vi "OpenDevices.vi"(7 "error In":errorcluster, 10 "Names":string[](array[string])) -> (0 "error out":errorcluster, 2 "Serial nos":u32[](array[numeric]), 3 "IDs":i32[](array[numeric]))   [LabVIEW 2020]
uses:
  libximc.lvlib
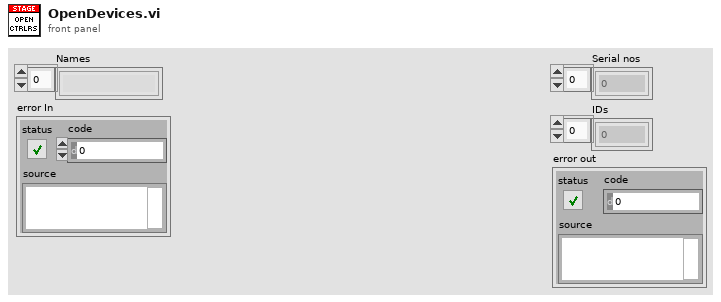
[diagram p1: front panel]
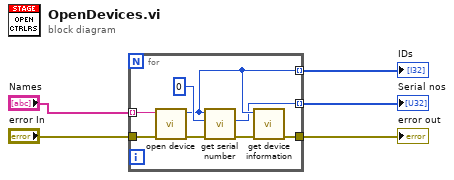
[diagram p0: block diagram]
diagram:
  n1 = for {
    tunnel: "error In" -> [w13]
    tunnel: [w6] -> w1
    tunnel: [w10] -> w2 mode=indexing
    tunnel: "Names" -> [w8] mode=indexing
    tunnel: [w7] -> w3 mode=indexing
    n2 = call "open device.vi"("error in (no error)"=w13, "uri"=w8) -> ("error out"=w9:errorcluster, "function return"=w10:i32)  [unwired: 8 in]
    n3 = call "get serial number.vi"("error in (no error)"=w9, "SerialNumber"=u32 0 ("serial"), "id"=w10) -> ("error out"=w11:errorcluster, "SerialNumber out"=w7:u32)  [unwired: 6 in, 1 out]
    n4 = call "get device information.vi"("error in (no error)"=w11, "id"=w10) -> ("error out"=w6:errorcluster)  [unwired: 7 in, 2 out]
  }
  "Serial nos" <- w3
  "IDs" <- w2
  "error out" <- w1
